vi "Main Screen 2.vi"() -> ()   [LabVIEW 2013]
uses:
  <vilib>/addons/_NISVFA/_Shared subVIs/Data Objects/Data/Data.lvclass
  <vilib>/addons/_NISVFA/_Shared subVIs/Data Objects/Y (DBL)/SV Convert Spectrum to Data Object.vi
  <vilib>/addons/_NISVFA/_Shared subVIs/Data Objects/Y (DBL)/Y (1 Ch).lvclass
panel:
  in  "RPM":enum32{"FFT", "CAN", "Sensor"}(radio)
  in  "AVT IP Address":dbl
  in  "CAN Addr.":dbl
  in  "CAN RPM Scale":dbl
  in  "CAN Low bit":dbl
  in  "CAN High bit":dbl
  in  "Sensor RPM Scale":dbl
  in  "High Frequency":dbl
  in  "Low Frequency":dbl
  in  "RPM +/-":dbl
  in  "pb.Calibration":bool
  in  "pb.RunScreen":bool
  in  "pb.StandConfig":bool
  in  "pb.TestConfig":bool
  in  "Tab Control":T1(tab)
  in  "Efficiency (%)":dbl
  in  "Speed (RPM)":dbl
  in  "Current (A)":dbl
  in  "Fuel Temp (C)":dbl
  in  "Plow (LpH)":dbl
  in  "Pressure (kPA)":dbl
  in  "Parameter 2":u16(ring) caption="ring.parameter2" items=["", "Voltage", "RPM", "Pressure", "Flow", "Deadhead"]
  in  "Parameter 1":u16(ring) caption="ring.parameter1" items=["", "Voltage", "RPM", "Pressure", "Flow", "Deadhead"]
  in  "Setpoint2":dbl caption="Pressure Setpoint"
  in  "Setpoint1":dbl caption="RPM Setpoint"
  in  "File Location":string
  in  "table.TestData":string[][](table)
  in  "pb.StopManual":bool
  in  "pb.StartManual":bool
  in  "pb.GrabData":bool
  in  "pb.StartTest":bool
  in  "pb.stats":bool
  in  "pb.trace":bool
  in  "pb.fft":bool
  in  "Voltage (DC)":dbl
  out "Stabilized?":bool
  in  "pb.load":bool
  in  "pb.save":bool
  in  "pb.new":bool
  in  "pb.run":bool
  in  "Parameter Information":string[][](table)
  in  "Model":string
  in  "Tank #":string
  in  "Fuel Batch #":string
  in  "Test Fluid":string
  in  "Durability Fluid":string
  in  "# of Comm Segs":string
  in  "Hours":string
  in  "Customer Ref#":string
  in  "Tracking #":string
  in  "Name":string
  in  "Serial Numbers":i32(listbox)
  out "Waveform Graph":dbl[](graph)
  in  "Max Voltage":dbl
  in  "Free Flow Pressure":dbl
  in  "Free Flow Voltage":dbl
  in  "Init Free Flow (sec)":dbl
  in  "Current Limit":dbl
  in  "Stable Count (sec)":dbl
  in  "Flow Tolerance":dbl
  in  "Voltage Tolerance":dbl
  in  "kPa Tolerance":dbl
  in  "Parameter Timeout (sec)":dbl
  in  "Max Flow":dbl
  in  "Min Flow":dbl
  in  "pb.saveFFT":bool
  # "Run Screen"
  # "Serial#?"
  # "Test Configuration Page"
  # "Stand Configuration Page"
  # "Calibration Page"
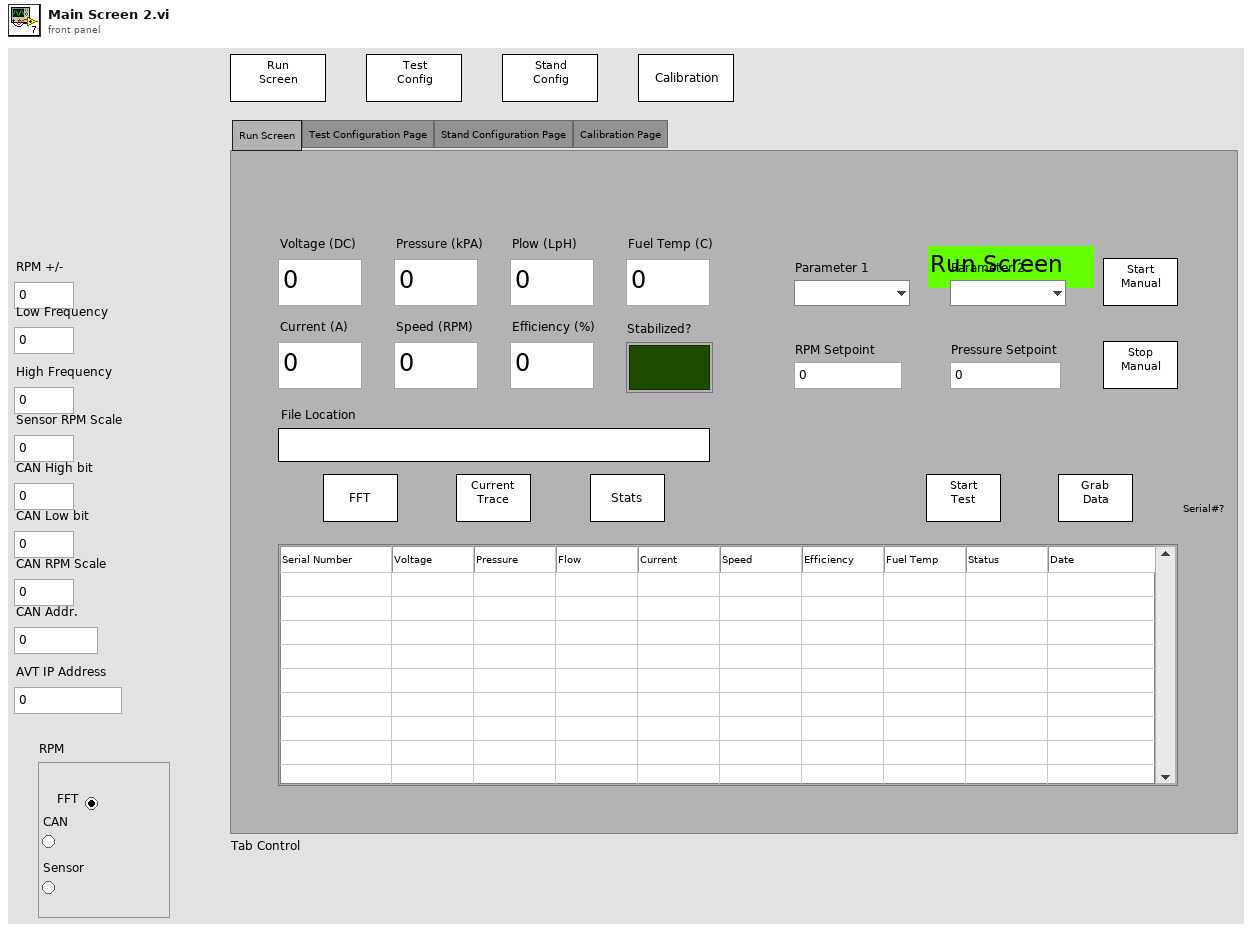
[diagram p1: front panel]
types:
  T1 = enum32{"Run Screen", "Test Configuration Page", "Stand Configuration Page", "Calibration Page"}
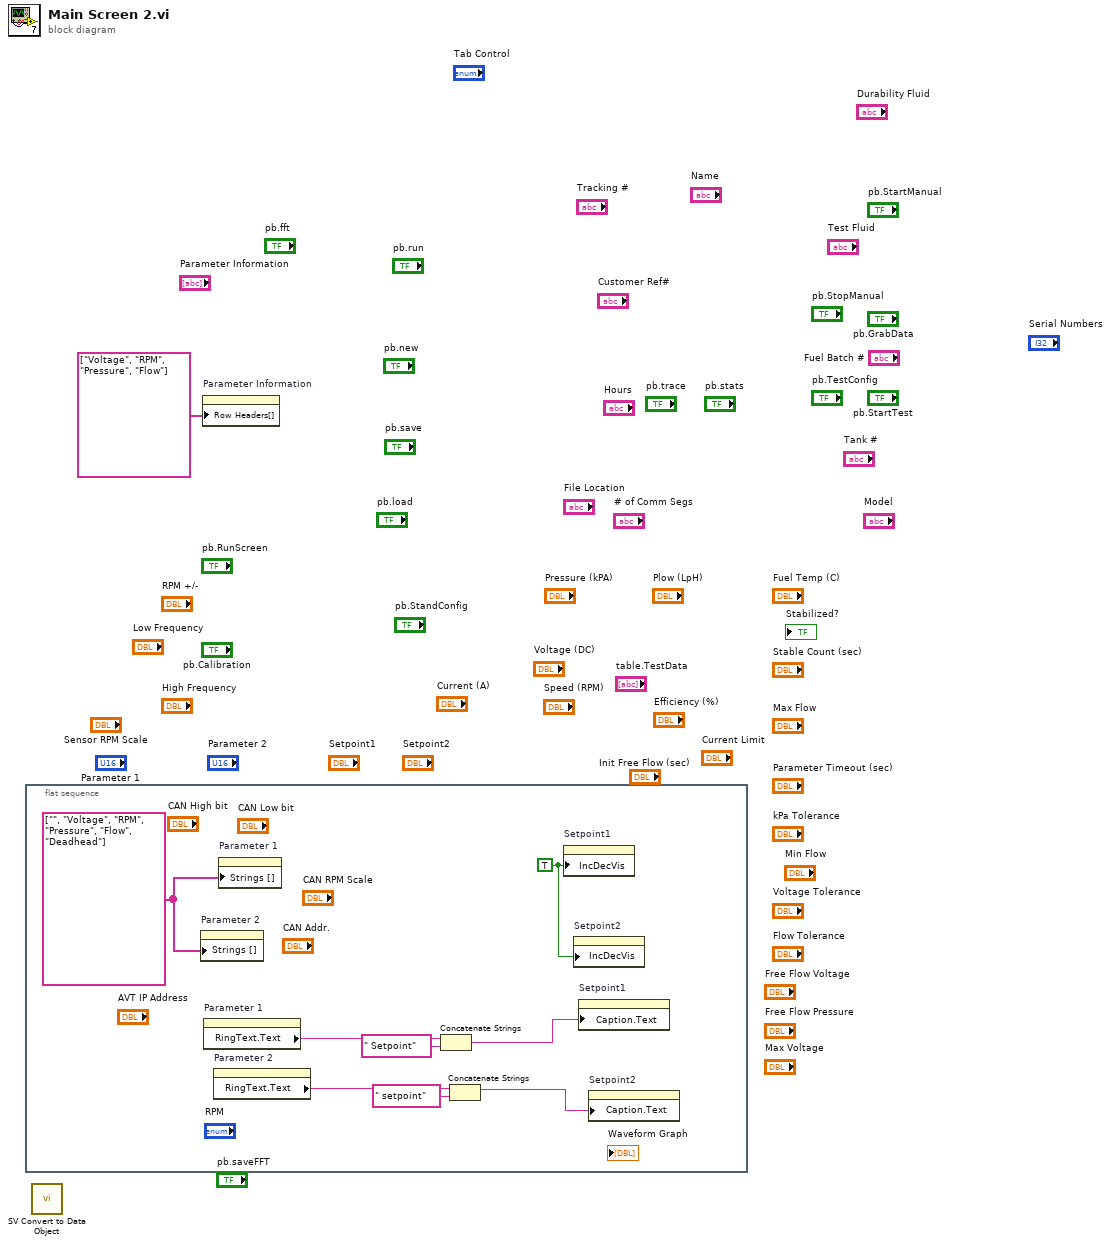
[diagram p0: block diagram]
diagram:
  n1 = flat-sequence {
    frame #0 {
      w9 = string[] ["", "Voltage", "RPM", "Pressure", "Flow", "Deadhead"]
      w10 = TRUE ("Increment/Decrement Visible?")
      n2 = property on="Parameter 2" class="Ring (strict)"("Strings []"=w9) -> ()  [unwired: 2 in, 2 out]
      n3 = property on="Parameter 1" class="Ring (strict)"() -> ("RingText.Text"=w7:string)  [unwired: 2 in, 2 out]
      n4 = property on="Parameter 2" class="Ring (strict)"() -> ("RingText.Text"=w8:string)  [unwired: 2 in, 2 out]
      n5 = property on="Parameter 1" class="Ring (strict)"("Strings []"=w9) -> ()  [unwired: 2 in, 2 out]
      n6 = Concatenate Strings(w7, " Setpoint" ("string")) -> (w6:string)
      n7 = Concatenate Strings(w8, " setpoint" ("string")) -> (w5:string)
      n8 = property on="Setpoint1" class="DigNum (strict)"("IncDecVis"=w10) -> ()  [unwired: 2 in, 2 out]
      n9 = property on="Setpoint2" class="DigNum (strict)"("IncDecVis"=w10) -> ()  [unwired: 2 in, 2 out]
      n10 = property on="Setpoint1" class="DigNum (strict)"("Caption.Text"=w6) -> ()  [unwired: 2 in, 2 out]
      n11 = property on="Setpoint2" class="DigNum (strict)"("Caption.Text"=w5) -> ()  [unwired: 2 in, 2 out]
    }
  }
  n12 = call-poly <vilib>:"SV Convert to Data Object.vi"() -> ("Spectrum Data"=w1:refnum<class "Data.lvclass">)  [unwired: 18 in, 1 out]
  n13 = property on="Parameter Information" class="Tbl (strict)"("Row Headers[]"=string[] ["Voltage", "RPM", "Pressure", "Flow"] ("Row Header Strings[]")) -> ()  [unwired: 2 in, 2 out]
